vi "Calc Impedance.vi"(10 "imp mode":bool, 11 "Array":dbl[](array[numeric])) -> (3 "Impedance":dbl)   [LabVIEW 2019, in "CML UI.lvlib"]
uses:
  CML UI.lvlib
  <vilib>/Analysis/3filter.llb/Filter Passband Type.ctl
  <vilib>/Analysis/baseanly.llb/Mean (DBL).vi
  <vilib>/Analysis/5stat.llb/RMS (DBL).vi
  <vilib>/Analysis/NI_AALBase.lvlib
  <vilib>/Analysis/NI_AALPro.lvlib
  <vilib>/ptbypt/NI_PtbyPt.lvlib
  <vilib>/Analysis/3filter.llb/Butterworth Filter (DBL).vi
panel:
  out "error":i32
  out "U. Impedance":dbl
  out "filtered Array":dbl[](graph)
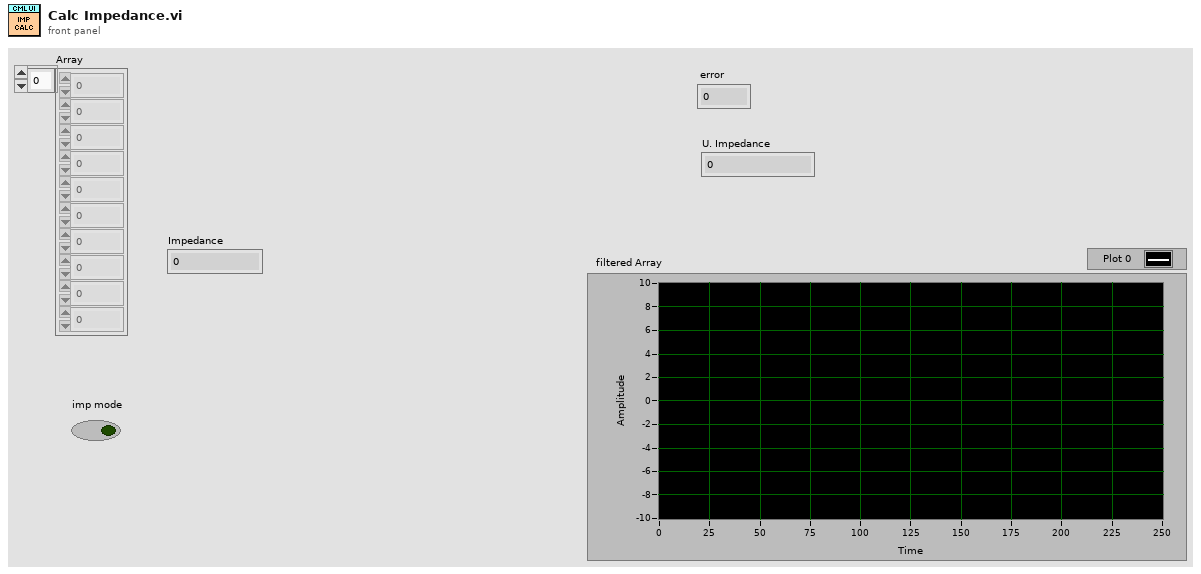
[diagram p1: front panel]
types:
  T1 = typedef "NI_AALBase.lvlib/Filter Passband Type.ctl" = enum32{"Lowpass", "Highpass", "Bandpass", "Bandstop"}
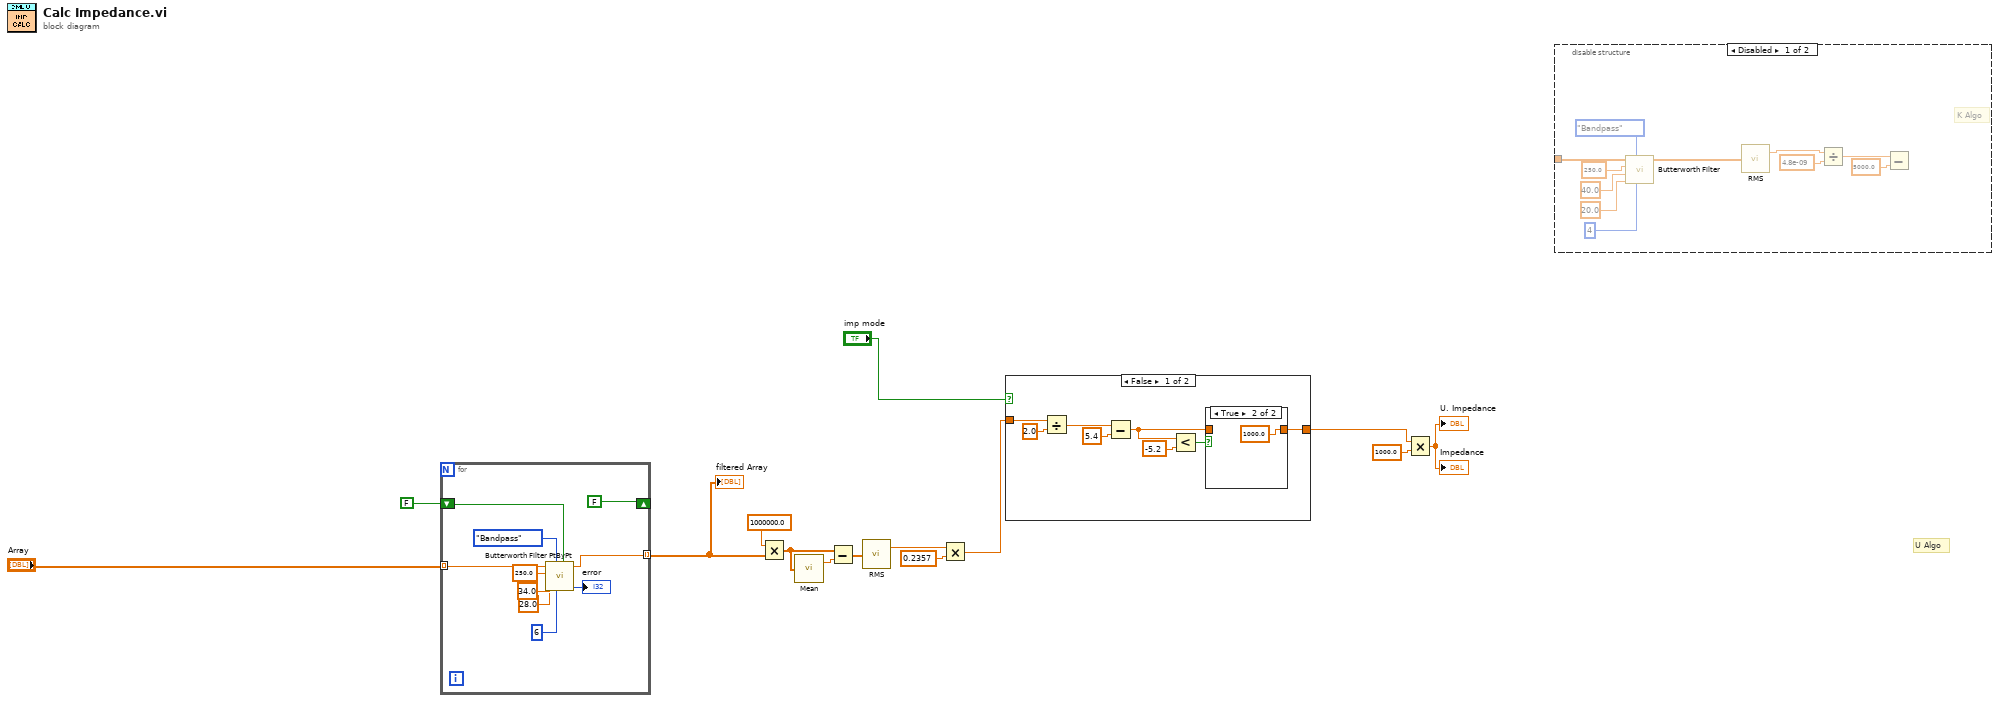
[diagram p0: block diagram]
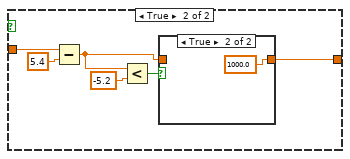
[diagram p3: hidden frame]
diagram:
  # "U Algo"
  n1 = for {
    tunnel: "Array" -> [w24] mode=indexing
    tunnel: [w23] -> w4 mode=indexing
    shift-right: [FALSE] -> _
    shift-left: FALSE -> [w21]
    n2 = call <vilib>:"Butterworth Filter PtByPt.vi"("initialize"=w21, "order"=6, "filter type"=Filter_Passband_Type."Bandpass", "low cutoff freq: fl"=28.0, "high cutoff freq: fh"=34.0, "sampling freq: fs"=250.0, "x"=w24) -> ("error"=→"error":i32, "Filtered x"=w23:dbl)  [unwired: 2 in]
  }
  "filtered Array" <- w4
  n3 = Multiply(x=1000000.0, y=w4) -> (x*y=w13:dbl[])
  n4 = call-poly <vilib>:"Mean.vi"("X"=w13) -> ("mean"=w12:dbl)  [unwired: 1 out]
  n5 = Subtract(x=w13, y=w12) -> (x-y=w11:dbl[])
  n6 = call-poly <vilib>:"RMS.vi"("X"=w11) -> ("rms value"=w10:dbl)  [unwired: 1 out]
  n7 = Multiply(x=w10, y=0.2357) -> (x*y=w3:dbl)
  n8 = case shown="False" "imp mode" {
    tunnel: w3 -> [w25 w39]
    tunnel: [w26 w36] -> w2
    frame False {
      n9 = Divide(x=w25, y=2.0) -> (x/y=w31:dbl)
      n10 = Subtract(x=w31, y=5.4 ("x")) -> (x-y=w28:dbl)
      n11 = Less?(x=w28, y=-5.2) -> (x < y?=w27:bool)
      n12 = case shown="True" w27 {
        tunnel: w28 -> [w33 _]
        tunnel: [w33 1000.0 ("y")] -> w26
        frame False {
        }
        frame True {
        }
      }
    }
    frame True {
      n13 = Subtract(x=w39, y=5.4 ("x")) -> (x-y=w37:dbl)
      n14 = Less?(x=w37, y=-5.2) -> (x < y?=w35:bool)
      n15 = case shown="True" w35 {
        tunnel: w37 -> [w41 _]
        tunnel: [w41 1000.0 ("y")] -> w36
        frame False {
        }
        frame True {
        }
      }
    }
  }
  n16 = Multiply(x=w2, y=1000.0) -> (x*y=→"Impedance" →"U. Impedance":dbl)
  n17 = disable-structure shown="Disabled" {
    disable-tunnel: _ -> [w53 _]
    frame Disabled {
      # "K Algo"
      n18 = call-poly <vilib>:"Butterworth Filter.vi"("order"=4, "filter type"=Filter_Passband_Type."Bandpass", "low cutoff freq: fl"=20.0, "high cutoff freq: fh"=40.0, "sampling freq: fs"=250.0, "X"=w53) -> ("Filtered X"=w43:dbl[])  [unwired: 2 in, 1 out]
      n19 = call-poly <vilib>:"RMS.vi"("X"=w43) -> ("rms value"=w52:dbl)  [unwired: 1 out]
      n20 = Divide(x=w52, y=4.8e-09) -> (x/y=w51:dbl)
      n21 = Subtract(x=w51, y=5000.0) -> ()  [unwired: 1 out]
    }
    frame Enabled {
    }
  }
